vi "Actor Core.vi"(8 "error in":errorcluster, 11 "POLARIS Target Focus Actor in":refnum<class "POLARIS Target Focus Actor.lvclass">) -> (0 "error out":errorcluster, 3 "Actor out":refnum<class "Actor.lvclass">)   [LabVIEW 2014, in "POLARIS Target Focus Actor.lvlib" / "POLARIS Target Focus Actor.lvclass"]
doc: "(<B>Filename</B>: Actor Framework.lvlib:Actor.lvclass:Actor Core.vi)\n\nReceives messages to the actor, reacts to them, and initiates any error handling that may shut the actor down.\n\nDescendant classes may override this VI to append parallel tasks for the actor to complete while it handles messages. Overrides use the Call Parent Method node."
uses:
  POLARIS Target Focus Actor.lvclass
  <vilib>/ActorFramework/Actor/Actor.lvclass
  Utility/Width Method.ctl
  IMAQdx Actor/IMAQdx Actor/IMAQdx Actor.lvclass
  HIJ Vision Display/HIJ Vision Display Messages/New Image Msg/New Image Msg.lvclass
  POLARIS Target Focus Actor Messages/New Results Msg/New Results Msg.lvclass
  POLARIS TA Focus Display/POLARIS TA Focus Display/POLARIS TA Focus Display.lvclass
  Analyze Parameter/Analyze Parameter Energy/Analyze Parameter Energy.lvclass
  Analyze Parameter/Analyze Parameter Width Method/Width Method.lvclass
  Analyze Parameter/Analyze Parameter Fluence/Analyze Parameter Fluence.lvclass
  Analyze Parameter/Analyze Parameter Energy/Analyze Parameter Energy.lvclass/Analyze Parameter Energy.ctl
  POLARIS Target Focus Actor.lvclass/POLARIS Target Focus Actor.ctl
  HIJ Vision Display/HIJ Vision Display/HIJ Vision Display.lvclass/HIJ Vision Display.ctl
  HIJ IMAQdx Display/AF IMAQ Display/HIJ IMAQdx Display.lvclass/HIJ IMAQdx Display.ctl
  Camera Actor/Camera Actor Messages/Start Acquisition Msg/Start Acquisition Msg.lvclass/Start Acquisition Msg.ctl
  <vilib>/ActorFramework/Message Enqueuer/Message Enqueuer.lvclass/Message Enqueuer.ctl
  Camera Actor/Camera Actor Messages/Write Receiver Params Msg/Write Receiver Params Msg.lvclass/Write Receiver Params Msg.ctl
  Shared Code/Viewable Actor/ViewableActor Messages/Insert Into SubPanel Msg/Insert Into SubPanel Msg.lvclass/Insert Into SubPanel Msg.ctl
  <vilib>/ActorFramework/Actor/Actor.lvclass/Actor.ctl
  HIJ Vision Display/HIJ Vision Display Messages/Write Image Name Prefix Msg/Write Image Name Prefix Msg.lvclass/Write Image Name Prefix Msg.ctl
  HIJ Vision Display/HIJ Vision Display Messages/Write WorkDir Msg/Write WorkDir Msg.lvclass/Write WorkDir Msg.ctl
  HIJ IMAQdx Display/AF IMAQ Display Messages/Write ConfigDir Msg/Write ConfigDir Msg.lvclass/Write ConfigDir Msg.ctl
  <vilib>/ActorFramework/Message Enqueuer/Message Priority.ctl
  POLARIS Target Focus Actor Messages/Start Sequence Msg/Start Sequence Msg.lvclass/Start Sequence Msg.ctl
  Analyze Parameter/Analyze Parameter Energy/Write Energy.vi
  HIJ Vision Display/HIJ Vision Display/Write Image Source Name.vi
  HIJ IMAQdx Display/AF IMAQ Display/Write ConfigDir.vi
  HIJ Vision Display/HIJ Vision Display/Write Save Report_.vi
  HIJ Vision Display/HIJ Vision Display/Write Show ZoomBtn_.vi
  HIJ Vision Display/HIJ Vision Display/Write WorkDir.vi
  HIJ Vision Display/HIJ Vision Display/Write Image Name Prefix.vi
  HIJ Vision Display/HIJ Vision Display/Write Publish Analyze Results Msg.vi
  <vilib>/ActorFramework/Message Enqueuer/Enqueue.vi
  <vilib>/ActorFramework/Message Enqueuer/Init from Existing Queue.vi
  <vilib>/ActorFramework/Message Priority Queue/Priority Enqueue.vi
  Camera Actor/Camera Actor Messages/Start Acquisition Msg/Start Acquisition Msg.lvclass
  Camera Actor/Camera Actor Messages/Write Receiver Params Msg/Write Receiver Params Msg.lvclass
  Shared Code/Viewable Actor/ViewableActor Messages/Insert Into SubPanel Msg/Insert Into SubPanel Msg.lvclass
  <vilib>/ActorFramework/Message Enqueuer/Message Enqueuer.lvclass
  <vilib>/ActorFramework/Stop Msg/Stop Msg.lvclass
  HIJ Vision Display/HIJ Vision Display Messages/Write Image Name Prefix Msg/Write Image Name Prefix Msg.lvclass
  HIJ Vision Display/HIJ Vision Display Messages/Write WorkDir Msg/Write WorkDir Msg.lvclass
  HIJ IMAQdx Display/AF IMAQ Display Messages/Write ConfigDir Msg/Write ConfigDir Msg.lvclass
  HIJ Vision Display/HIJ Vision Display Messages/Save Image Msg/Save Image Msg.lvclass
  POLARIS Target Focus Actor Messages/Stop Sequence Msg/Stop Sequence Msg.lvclass
  POLARIS Target Focus Actor Messages/Start Sequence Msg/Start Sequence Msg.lvclass
  Utility/POLARIS Vision utility.lvlib
panel:
  out "Act Seq Nr":u16 caption="ImgNr."
  in  "Results String":string
  in  "#to save":u16=10
  in  "Save Seq":bool
  in  "Stop Signal":bool
  in  "Save":bool
  in  "Image Prefix":string
  out "q-Factor":dbl format="%#_3g"
  out "Focus/µm^2":dbl format="%#.1g"
  out "I [W/cm^2]":dbl format="%#.2g"
  in  "WorkDir":path
  in  "Config Dir":path
  in  "Energy":dbl[unit]=10.0
  in  "Size of hot Region":i32=10
  in  "Method":T1
  in  "Camera Name":string
  in  "Pulse duration [fs]":dbl=150.0
  in  "Compressor eff.":dbl=0.63
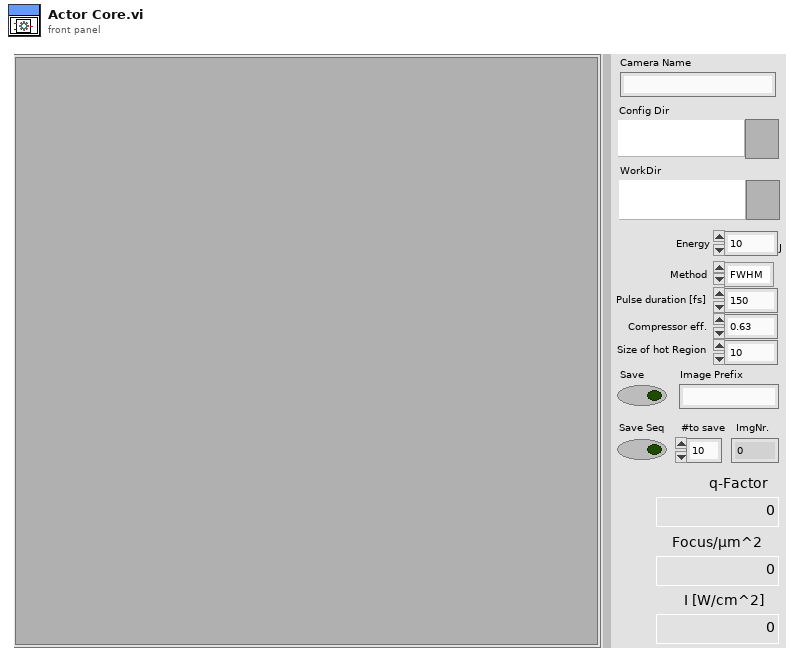
[diagram p1: front panel]
types:
  T1 = typedef "POLARIS Vision utility.lvlib/Width Method.ctl" = enum16{"FWHM", "1/e", "1/e^2", "80%", "90%"}
  T2 = typedef "Actor Framework.lvlib/Message Enqueuer.lvclass/Message Priority.ctl" = enum16{"Low", "Normal", "High"}
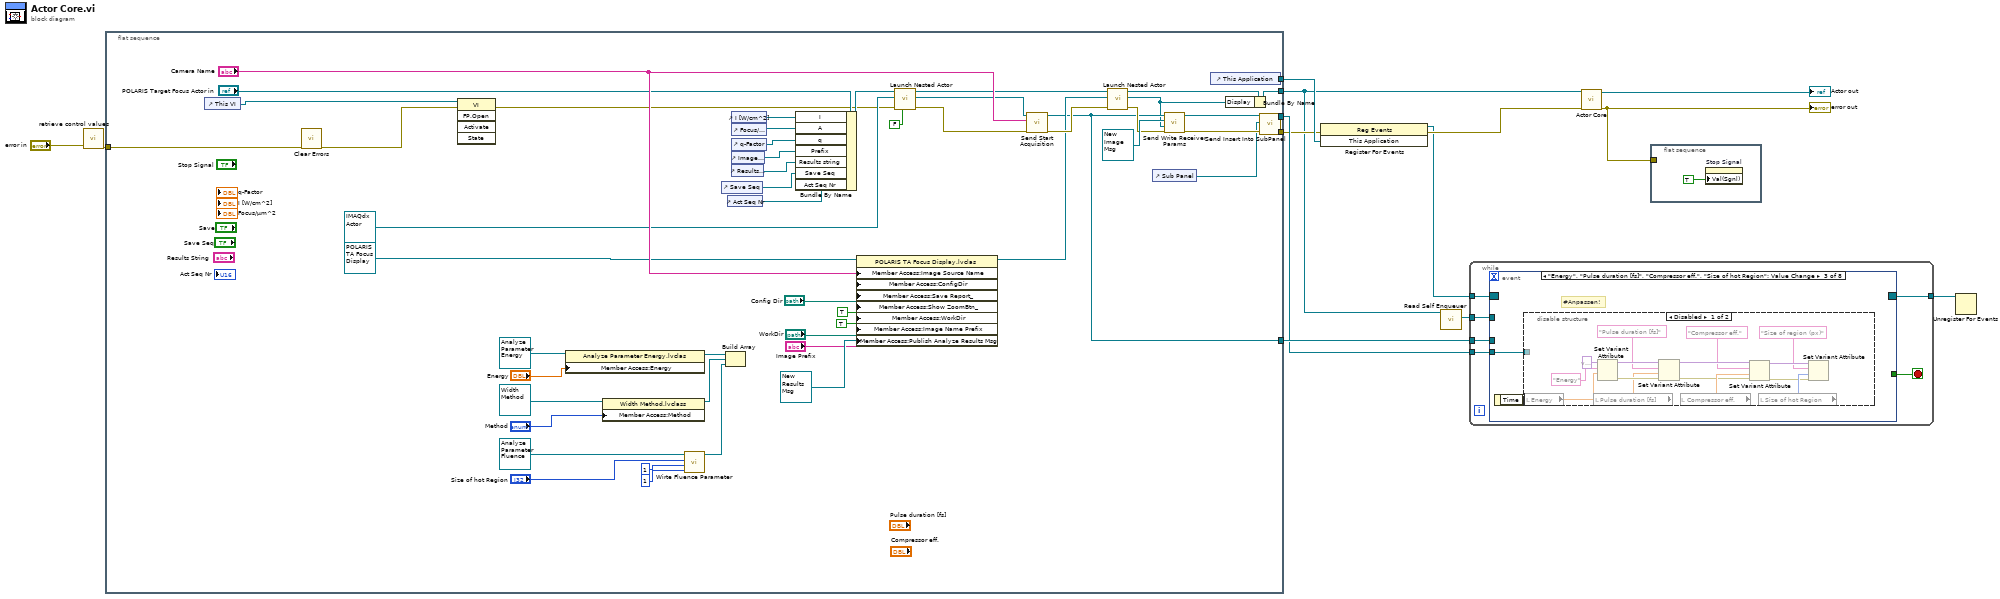
[diagram p0: block diagram]
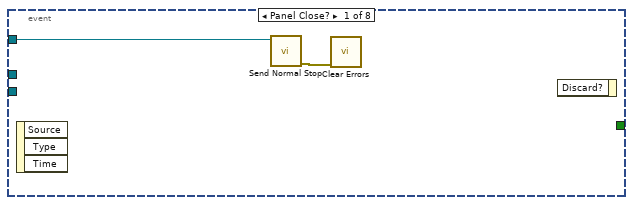
[diagram p2: hidden frame]
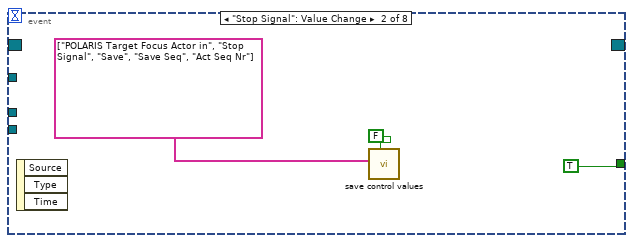
[diagram p3: hidden frame]
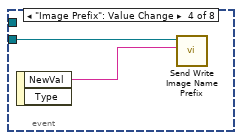
[diagram p5: hidden frame]
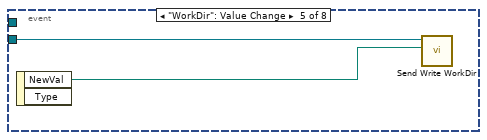
[diagram p6: hidden frame]
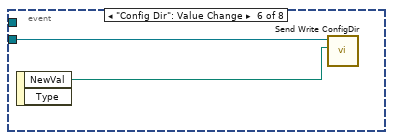
[diagram p7: hidden frame]
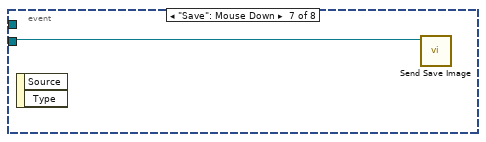
[diagram p8: hidden frame]
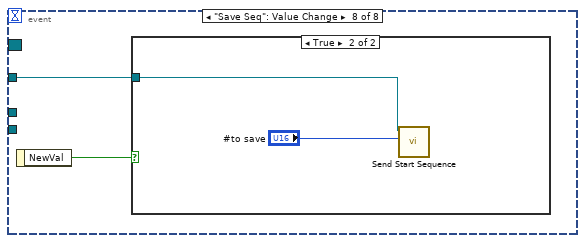
[diagram p9: hidden frame]
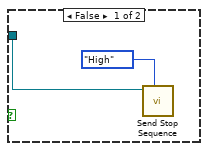
[diagram p10: hidden frame]
diagram:
  n1 = call "retrieve control values.vi"("error in (no error)"="error in") -> ("error out"=w13:errorcluster)  [unwired: 9 in, 1 out]
  n2 = flat-sequence {
    tunnel: w13 -> [w64]
    tunnel: [w48] -> w10
    tunnel: [w47] -> w9
    tunnel: [w37] -> w6
    tunnel: [w36] -> w5
    tunnel: [w31] -> w1
    frame #0 {
      n3 = control-ref of="This VI"() -> (w60:refnum<vi>)
      n4 = call <vilib>:"Clear Errors.vi"("error in (no error)"=w64) -> ("error out"=w32:errorcluster)  [unwired: 5 in, 1 out]
      n5 = invoke class="VI" method="FP.Open"(reference=w60, error in=w32) -> (error out=w33:errorcluster)  [unwired: 3 in, 4 out]
      n6 = property class="Analyze Parameter Energy.lvclas"(reference=refnum<class "Analyze Parameter Energy.lvclass"> refnum ("Analyze Parameter Energy.lvclass"), "Member Access:Energy"="Energy") -> (reference out=w16:refnum<class "Analyze Parameter Energy.lvclass">)  [unwired: 1 in, 1 out]
      n7 = property class="Width Method.lvclass"(reference=refnum<class "Width Method.lvclass"> refnum ("Width Method.lvclass"), "Member Access:Method"="Method") -> (reference out=w15:refnum<class "Width Method.lvclass">)  [unwired: 1 in, 1 out]
      n8 = call "Wirte Fluence Parameter.vi"("#of Areas"=1, "#Overlays"=1, "Size of region (px)"="Size of hot Region", "Analyze Parameter Fluence in"=refnum<class "Analyze Parameter Fluence.lvclass"> refnum ("Analyze Parameter Fluence.lvclass")) -> ("Analyze Parameter Fluence out"=w14:refnum<class "Analyze Parameter Fluence.lvclass">)  [unwired: 7 in]
      n9 = control-ref of="Save Seq"() -> (w28:refnum<vi>)
      n10 = Build Array(w16, w15, w14) -> ()  [unwired: 1 out]
      n11 = control-ref of="Act Seq Nr"() -> (w27:refnum<vi>)
      n12 = control-ref of="I [W/cm^2]"() -> (w40:refnum<vi>)
      n13 = control-ref of="Focus/µm^2"() -> (w39:refnum<vi>)
      n14 = control-ref of="Results String"() -> (w34:refnum<vi>)
      n15 = control-ref of="q-Factor"() -> (w38:refnum<vi>)
      n16 = control-ref of="Image Prefix"() -> (w35:refnum<vi>)
      n17 = Bundle By Name(cluster="POLARIS Target Focus Actor in", "I"=w40, "A"=w39, "q"=w38, "Prefix"=w35, "Results string"=w34, "Save Seq"=w28, "Act Seq Nr"=w27) -> (w41:refnum<class "POLARIS Target Focus Actor.lvclass">)
      n18 = property class="POLARIS TA Focus Display.lvclas"(reference=refnum<class "POLARIS TA Focus Display.lvclass"> refnum ("POLARIS TA Focus Display.lvlib:POLARIS TA Focus Display.lvclass"), "Member Access:Image Source Name"="Camera Name", "Member Access:ConfigDir"="Config Dir", "Member Access:Save Report_"=TRUE ("Save Report_"), "Member Access:Show ZoomBtn_"=TRUE ("Show ZoomBtn_"), "Member Access:WorkDir"="WorkDir", "Member Access:Image Name Prefix"="Image Prefix", "Member Access:Publish Analyze Results Msg"=refnum<class "New Results Msg.lvclass"> refnum ("POLARIS Target Focus Actor.lvlib:New Results Msg.lvclass")) -> (reference out=w50:refnum<class "POLARIS TA Focus Display.lvclass">)  [unwired: 1 in, 1 out]
      n19 = call <vilib>:"Launch Nested Actor.vi"("Open Actor Core front panel? (F)"=FALSE, "error in (no error)"=w33, "Nested Actor"=refnum<class "IMAQdx Actor.lvclass"> refnum ("IMAQdx Actor.lvlib:IMAQdx Actor.lvclass"), "Caller Actor in"=w41) -> ("error out"=w59:errorcluster, "Nested Actor's Enqueuer"=w58:refnum<class "Message Enqueuer.lvclass">, "Caller Actor out"=w54:refnum<class "POLARIS Target Focus Actor.lvclass">)  [unwired: 5 in]
      n20 = call "Send Start Acquisition.vi"("error in (no error)"=w59, "Camera Name"="Camera Name", "Message Enqueuer"=w58) -> ("error out"=w52:errorcluster, "Message Enqueuer out"=w48:refnum<class "Message Enqueuer.lvclass">)  [unwired: 7 in]
      n21 = call <vilib>:"Launch Nested Actor.vi"("error in (no error)"=w52, "Nested Actor"=w50, "Caller Actor in"=w54) -> ("error out"=w51:errorcluster, "Nested Actor's Enqueuer"=w30:refnum<class "Message Enqueuer.lvclass">, "Caller Actor out"=w53:refnum<class "POLARIS Target Focus Actor.lvclass">)  [unwired: 6 in]
      n22 = control-ref of="Sub Panel"() -> (w45:refnum<vi>)
      n23 = call "Send Write Receiver Params.vi"("error in (no error)"=w51, "Image Receiver"=w30, "New Image Msg"=refnum<class "New Image Msg.lvclass"> refnum ("AF IMAQ Display.lvlib:New Image Msg.lvclass"), "Message Enqueuer"=w48) -> ("error out"=w56:errorcluster, "Message Enqueuer out"=w49:refnum<class "Message Enqueuer.lvclass">)  [unwired: 6 in]
      n24 = control-ref of="This Application"() -> (w37:refnum<vi>)
      n25 = Bundle By Name(cluster=w53, "Display"=w30) -> (w31:refnum<class "POLARIS Target Focus Actor.lvclass">)
      n26 = call "Send Insert Into SubPanel.vi"("error in (no error)"=w56, "SubPanel Ref"=w45, "Message Enqueuer"=w49) -> ("error out"=w36:errorcluster, "Message Enqueuer out"=w47:refnum<class "Message Enqueuer.lvclass">)  [unwired: 7 in]
    }
  }
  n27 = register-events(error in=w5, w6) -> (reference out=w3:refnum<event-registration>, error out=w4:errorcluster)  [unwired: 1 in]
  n28 = call <vilib>:"Read Self Enqueuer.vi"("Actor"=w1) -> ("Self Enqueuer"=w11:refnum<class "Message Enqueuer.lvclass">)  [unwired: 10 in]
  n29 = while {
    tunnel: w11 -> [w69]
    tunnel: w10 -> [w68]
    tunnel: w9 -> [w67]
    tunnel: w3 -> [w66]
    tunnel: [w65] -> w2
    stop <- w70 stop-if-true
    n30 = event shown="[2] \"Energy\", \"Pulse duration [fs]\", \"Compressor eff.\", \"Size of hot Region\": Value Change" {
      selector: w66 -> [_ _ _ _ _ _ _ _]
      dyn-events: [_ _ _ _ _ _ _ _] -> w65
      timeout: _ -> [_ _ _ _ _ _ _ _]
      tunnel: [_ TRUE _ _ _ _ _ _] -> w70
      tunnel: w69 -> [w72 _ _ _ _ _ _ w101]
      tunnel: w68 -> [_ _ _ _ _ _ _ _]
      tunnel: w67 -> [_ _ w76 w95 w97 w99 w100 _]
      event Panel Close? {
        n31 = event-data() -> ()  [unwired: 1 in, 3 out]
        n32 = call <vilib>:"Send Normal Stop.vi"("Message Enqueuer"=w72) -> ("error out"=w71:errorcluster)  [unwired: 10 in]
        n33 = call <vilib>:"Clear Errors.vi"("error in (no error)"=w71) -> ()  [unwired: 5 in, 2 out]
        n34 = event-data() -> ()  [unwired: 2 in, 1 out]
      }
      event "Stop Signal": Value Change {
        n35 = event-data() -> ()  [unwired: 1 in, 3 out]
        n36 = call "save control values.vi"("Append timestamp (true)"=FALSE, "Dont save"=string[] ["POLARIS Target Focus Actor in", "Stop Signal", "Save", "Save Seq", "Act Seq Nr"]) -> ()  [unwired: 6 in, 2 out]
      }
      event "Energy", "Pulse duration [fs]", "Compressor eff.", "Size of hot Region": Value Change {
        # "#Anpassen!"
        n37 = event-data() -> ()  [unwired: 1 in, 1 out]
        n38 = disable-structure shown="Disabled" {
          disable-tunnel: w76 -> [w78 _]
          frame Disabled {
            n39 = local read "Energy"() -> (w89:dbl[unit])
            n40 = local read "Pulse duration [fs]"() -> (w86:dbl)
            n41 = Set Variant Attribute(Variant=variant ("variant"), name="Energy", value=w89) -> (Variant out=w85:variant, error out=w87:errorcluster)  [unwired: 1 in, 1 out]
            n42 = Set Variant Attribute(Variant=w85, name="Pulse duration [fs]", value=w86, error in=w87) -> (Variant out=w83:variant, error out=w82:errorcluster)  [unwired: 1 out]
            n43 = local read "Compressor eff."() -> (w88:dbl)
            n44 = Set Variant Attribute(Variant=w83, name="Compressor eff.", value=w88, error in=w82) -> (Variant out=w91:variant, error out=w92:errorcluster)  [unwired: 1 out]
            n45 = local read "Size of hot Region"() -> (w93:i32)
            n46 = Set Variant Attribute(Variant=w91, name="Size of region (px)", value=w93, error in=w92) -> (Variant out=w77:variant)  [unwired: 2 out]
          }
          frame Enabled {
          }
        }
      }
      event "Image Prefix": Value Change {
        n47 = event-data() -> ("NewVal"=w94:string)  [unwired: 1 in, 1 out]
        n48 = call "Send Write Image Name Prefix.vi"("Image Name Prefix"=w94, "Message Enqueuer"=w95) -> ()  [unwired: 8 in, 2 out]
      }
      event "WorkDir": Value Change {
        n49 = event-data() -> ("NewVal"=w96:path)  [unwired: 1 in, 1 out]
        n50 = call "Send Write WorkDir.vi"("WorkDir"=w96, "Message Enqueuer"=w97) -> ()  [unwired: 8 in, 2 out]
      }
      event "Config Dir": Value Change {
        n51 = event-data() -> ("NewVal"=w98:path)  [unwired: 1 in, 1 out]
        n52 = call "Send Write ConfigDir.vi"("ConfigDir"=w98, "Message Enqueuer"=w99) -> ()  [unwired: 8 in, 2 out]
      }
      event "Save": Mouse Down {
        n53 = event-data() -> ()  [unwired: 1 in, 2 out]
        n54 = call "Send Save Image.vi"("Message Enqueuer"=w100) -> ()  [unwired: 9 in, 2 out]
      }
      event "Save Seq": Value Change {
        n55 = event-data() -> ("NewVal"=w102:bool)  [unwired: 1 in]
        n56 = case shown="True" w102 {
          tunnel: w101 -> [w104 w106]
          frame False {
            n57 = call "Send Stop Sequence.vi"("Message Priority (Normal)"=Message_Priority."High", "Message Enqueuer"=w104) -> ()  [unwired: 8 in, 2 out]
          }
          frame True {
            n58 = call "Send Start Sequence.vi"("#to save"="#to save", "Message Enqueuer"=w106) -> ()  [unwired: 8 in, 2 out]
          }
        }
      }
    }
  }
  n59 = call-parent "Actor Core.vi"("error in"=w4, "Actor in"=w1) -> ("error out"=w7:errorcluster, "Actor out"=→"Actor out":refnum<class "Actor.lvclass">)  [unwired: 8 in]
  "error out" <- w7
  n60 = flat-sequence {
    tunnel: w7 -> [_]
    frame #0 {
      n61 = property on="Stop Signal" class="Bool (strict)"("Val(Sgnl)"=TRUE) -> ()  [unwired: 2 in, 2 out]
    }
  }
  n62 = Unregister For Events(event registration refnum=w2) -> ()  [unwired: 1 in, 1 out]
